vi "与或.vi"() -> ()   [LabVIEW 2018]
panel:
  out "或结果":bool
  out "与结果":bool
  in  "布尔 2":bool
  in  "布尔":bool
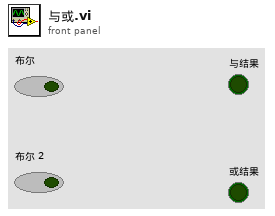
[diagram p1: front panel]
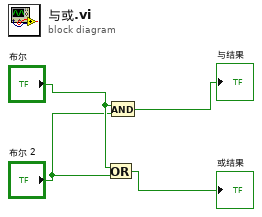
[diagram p0: block diagram]
diagram:
  n1 = Or(x="布尔", y="布尔 2") -> (x .or. y?=→"或结果":bool)
  n2 = And(x="布尔", y="布尔 2") -> (x .and. y?=→"与结果":bool)
